vi "Modbus Dialog Messages.vi"() -> ()   [LabVIEW 2013, in "Modbus Shared.lvlib"]
uses:
  Shared/Modbus Shared.lvlib
panel:
  in  "Confirmation to erase all existing channels":string="Content of Modbus Configuration File has changed. \nClick \"Continue\" to delete all existing Custom-Device Channels and create new Channels matching Configuration File.\nClick \"Cancel\" to keep existing Configuration."
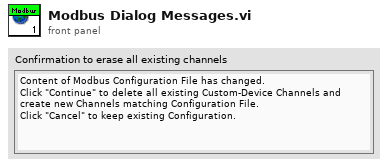
[diagram p1: front panel]
diagram:
